vi "unit_test.vi"(8 "error in (no error)":errorcluster) -> (0 "error out":errorcluster)   [LabVIEW 2019]
uses:
  <vilib>/addons/_JKI Toolkits/Caraya/classes/Assert/Assert Equal Value and Type_Variant.vi
  <vilib>/addons/_JKI Toolkits/Caraya/classes/Test/Test.lvclass
  <vilib>/addons/_JKI Toolkits/Caraya/classes/Assert/Assert.lvclass
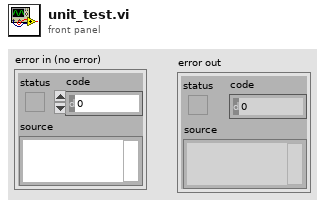
[diagram p1: front panel]
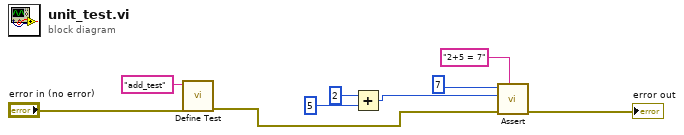
[diagram p0: block diagram]
diagram:
  n1 = call <vilib>:"Define Test.vi"("error in (no error)"="error in (no error)", "Label (VI Title)"="add_test") -> ("error out"=w3:errorcluster)  [unwired: 9 in]
  n2 = Add(x=2, y=5 ("x")) -> (x+y=w6:i32)
  n3 = call-poly <vilib>:"Assert.vi"("Label"="2+5 = 7", "error in (no error)"=w3, "Y"=w6, "X"=7 ("x")) -> ("error out"=→"error out":errorcluster)  [unwired: 7 in]
